vi "Initialize.vi"(8 "error in":errorcluster, 10 "shared resources":refnum<class "Shared Resources.lvclass">, 11 "Execution Unit Implementation in":refnum<class "Execution Unit.lvclass">) -> (0 "error out":errorcluster, 3 "Execution Unit Implementation out":refnum<class "Execution Unit.lvclass">)   [LabVIEW 2024, in "AIM ARINC 429 Engine.lvlib" / "Implementation.lvlib" / "Execution Unit.lvclass"]
uses:
  Execution Unit.lvclass
  Interfaces/Shared Resources/Shared Resources.lvclass
  Shared Resources/Shared Resources.lvclass
  Shared Resources/Shared Resources.lvclass/Shared Resources.ctl
  Execution Unit.lvclass/Execution Unit.ctl
  Shared Resources/Read board handle.vi
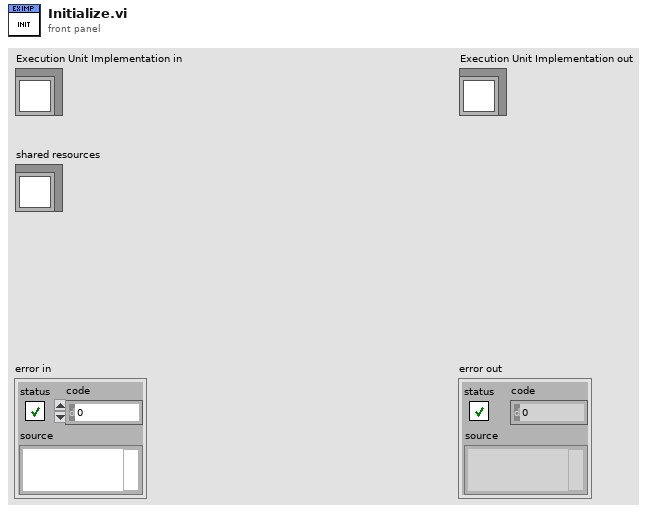
[diagram p1: front panel]
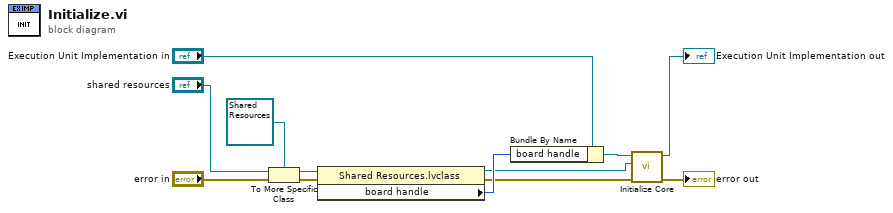
[diagram p0: block diagram]
diagram:
  n1 = To More Specific Class(target class=refnum<class "Shared Resources.lvclass"> refnum ("Shared Resources"), reference="shared resources", error in="error in") -> (specific class reference=w8:refnum<class "Shared Resources.lvclass">, error out=w9:errorcluster)
  n2 = property class="Shared Resources.lvclass"(reference=w8, error in=w9) -> (reference out=w1:refnum<class "Shared Resources.lvclass">, error out=w5:errorcluster, "board handle"=w6:u8)
  n3 = Bundle By Name(cluster="Execution Unit Implementation in", "board handle"=w6) -> (w3:refnum<class "Execution Unit.lvclass">)
  n4 = call-dynamic "Initialize Core.vi"("error in"=w5, "Shared Resources"=w1, "Execution Unit in"=w3) -> ("error out"=→"error out":errorcluster, "Execution Unit out"=→"Execution Unit Implementation out":refnum<class "Execution Unit.lvclass">)  [unwired: 7 in]
